vi "Measurement Logic.vi"() -> ()   [LabVIEW 2022 SP3, in "Single Tone - Digital Mic.lvlib"]
uses:
  Single Tone - Digital Mic.lvlib
  <vilib>/Plug-In SDKs/Measurements/Measure Call Context/Measure Call Context.lvclass
  Measurement Configuration.ctl
  shared/measurements/controls/lowpass filter.ctl
  shared/measurements/controls/weighting filter.ctl
  shared/measurements/controls/highpass filter.ctl
  shared/measurements/controls/measurement units.ctl
  Measurement Results.ctl
  <vilib>/addons/_NISVFA/_Generation/Signal Generation/SV Signal/sv_System Timing Model.ctl
  shared/Stop Variable Action.ctl
  <vilib>/PDM Acquisition Toolkit/host/Classes/Tasks/PDM Tasks/Controls/Acquisition Mode.ctl
  <vilib>/PDM Acquisition Toolkit/shared/controls/clock mode.ctl
  shared/measurements/controls/audio filter settings.ctl
  shared/measurements/controls/single tone microphone measurement settings.ctl
  shared/measurements/controls/units settings - mic.ctl
  <vilib>/DAQmx/read.llb/DAQmx Read (Analog Wfm 1Chan NSamp).vi
  <vilib>/DAQmx/write.llb/DAQmx Write (Analog Wfm 1Chan NSamp).vi
  <vilib>/addons/_NISVFA/_Generation/Signal Generation/SV Sinusoid/SV Sinusoid.lvclass
  C:/Program Files/NI/LVAddons/nisvt/1/vi.lib/addons/_NISVFA/_Generation/Signal Generation/SV Signal/SV Signal.lvclass
  <vilib>/addons/_NISVFA/_Generation/Signal Generation/SV Sinusoid/Configure Sine.vi
  <vilib>/DAQmx/create/channels.llb/DAQmx Create Channel (AO-Voltage-Basic).vi
  <vilib>/DAQmx/configure/timing.llb/DAQmx Timing (Sample Clock).vi
  <vilib>/DAQmx/configure/events/hardwareSignals.llb/DAQmx Export Signal (Most Signals).vi
  <vilib>/addons/_NISVFA/_Generation/Signal Generation/SV Signal/Write Sample Rate.vi
  <vilib>/addons/_NISVFA/_Generation/Signal Generation/SV Signal/Write System Timing Model.vi
  <vilib>/addons/_NISVFA/_Generation/Signal Generation/SV Signal/Write Ramp Parameters.vi
  <vilib>/DAQmx/create/channels.llb/DAQmx Create Channel (AI-Sound Pressure-Microphone).vi
  <vilib>/Waveform/WDTOps.llb/WDT Waveform Duration DBL.vi
  <vilib>/DAQmx/configure/trigger.llb/DAQmx Start Trigger (Digital Edge).vi
  <vilib>/DAQmx/miscellaneous.llb/DAQmx Fill In Error Info.vi
  <vilib>/Waveform/WDTOps.llb/WDT Get Waveform Subset DBL.vi
  <vilib>/addons/_NISVFA/_Generation/Signal Generation/SV Signal/SV Signal.lvclass
  <resource>/objmgr/daqmx.rc
  shared/combined digital api/Combo Digital Audio API.lvlib
  <vilib>/PDM Acquisition Toolkit/host/Classes/Tasks/PDM Tasks/PDM Task.lvclass
  <vilib>/PDM Acquisition Toolkit/shared/PDM Shared.lvlib
panel:
  out "calculated microphone sensitivity (dBFS)":dbl
  out "measurement results":T1={"channel name"="Empty", "frequency (Hz)"=0.0, "amplitude (Pa RMS)"=0.0, "amplitude (dBSPL)"=0.0, "microphone sensitivity (dBFS)"=0.0, "SNR"=0.0, "THD+N"=0.0, "THD"=0.0, "wfm - dt"=0.0, "wfm - data"=[0.0], "fft - f0"=0.0, "fft - df"=0.0, "fft - data"=[0.0], "ref mic wfm - dt"=0.0, "ref mic wfm - data"=[0.0]}
  in  "measurement configuration":T2={"digital channel list"="Lorem ipsum dolor sit", "input cfg file"="", "digital mic sensitivity (dBFS)"=1.2, "ref mic channel"="7821\\PCMo 0", "ref mic sensitivity (mV/Pa)"=32.0, "output channel"="7821\\PCMo 0", "signal frequency"=64.0, "output level (dBSPL)"=-32.0, "output voltage ratio"=-64.0, "lowpass filter"=enum."No filter", "weighting filter"=enum."A-weighting", "highpass filter"=enum."AC", "band start"=1.0, "band stop"=1.0, "min measurement cycles"=20, "min measurement time (s)"=0.1, "min settling cycles"=0, "min settling time (s)"=0.0, "SNR units"=enum."dB", "THD+N units"=enum."dB", "THD units"=enum."dB"} {"output voltage ratio" format="%#_g Pa/V"; "signal frequency" format="%#_13g"; "digital mic sensitivity (dBFS)" format="%#_13g"}
  out "measure call context out":refnum<class "Measure Call Context.lvclass">
  in  "measure call context in":refnum<class "Measure Call Context.lvclass">
  out "error out":errorcluster
  in  "error in":errorcluster
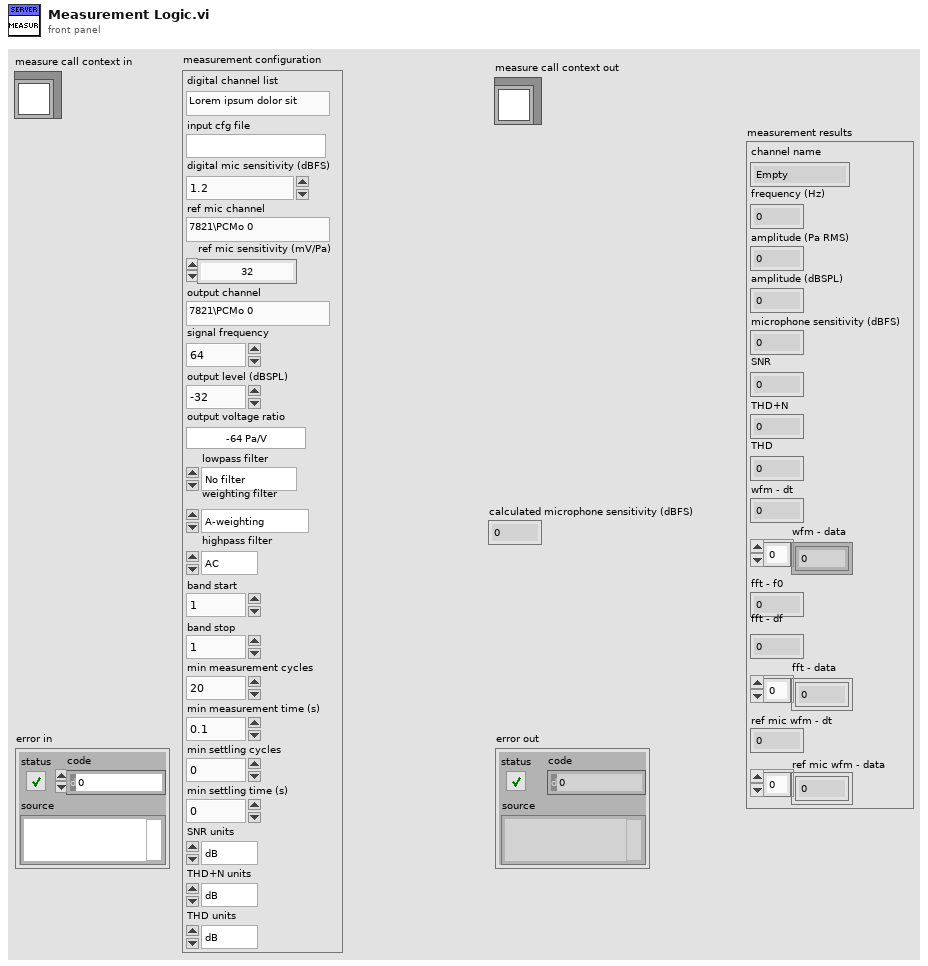
[diagram p1: front panel]
types:
  T1 = typedef "Single Tone - Digital Mic.lvlib/Measurement Results.ctl" = cluster{"channel name":string, "frequency (Hz)":dbl, "amplitude (Pa RMS)":dbl, "amplitude (dBSPL)":dbl, "microphone sensitivity (dBFS)":dbl, "SNR":dbl, "THD+N":dbl, "THD":dbl, "wfm - dt":dbl, "wfm - data":dbl[], "fft - f0":dbl, "fft - df":dbl, "fft - data":dbl[], "ref mic wfm - dt":dbl, "ref mic wfm - data":dbl[]}
  T2 = typedef "Single Tone - Digital Mic.lvlib/Measurement Configuration.ctl" = cluster{"digital channel list":string, "input cfg file":string, "digital mic sensitivity (dBFS)":dbl, "ref mic channel":string, "ref mic sensitivity (mV/Pa)":dbl, "output channel":string, "signal frequency":dbl, "output level (dBSPL)":dbl, "output voltage ratio":dbl, "lowpass filter":T3, "weighting filter":T4, "highpass filter":T5, "band start":dbl, "band stop":dbl, "min measurement cycles":u32, "min measurement time (s)":dbl, "min settling cycles":u32, "min settling time (s)":dbl, "SNR units":T6, "THD+N units":T6, "THD units":T6}
  T3 = typedef "lowpass filter.ctl" = enum32{"No filter", "AES17 20kHz", "AES17 40kHz"}
  T4 = typedef "weighting filter.ctl" = enum32{"Linear", "A-weighting", "B-weighting", "C-weighting"}
  T5 = typedef "highpass filter.ctl" = enum32{"DC", "AC"}
  T6 = typedef "measurement units.ctl" = enum32{"dB", "%", "x/y"}
  T7 = typedef "units settings - mic.ctl" = cluster{"SNR units":T6, "THD+N units":T6, "THD units":T6}
  T8 = typedef "single tone microphone measurement settings.ctl" = cluster{"Band start":dbl, "Band stop":dbl, "Frequency":dbl}
  T9 = typedef "audio filter settings.ctl" = cluster{"weighting filter":T4, "highpass filter":T5, "lowpass filter ":T3}
  T10 = typedef "PDM Shared.lvlib/clock mode.ctl" = enum16{"divided clock", "DDS"}
  T11 = typedef "PDM Acquisition Class Library.lvlib/PDM Task.lvclass/Acquisition Mode.ctl" = enum16{"Finite", "Continuous"}
  T12 = typedef "Stop Variable Action.ctl" = enum16{"Reset", "Check", "Stop"}
  T13 = typedef "SV Signal.lvclass/sv_System Timing Model.ctl" = i64
  T14 = cluster{"profile":enum16{"Linear", "Half cosine"}, "durations [s]":cluster{"ramp-up":dbl, "transition":dbl, "ramp-down":dbl}}
  T15 = typedef "Combo Digital Audio API.lvlib/task.ctl" = cluster{"task ref":u64, "audio type":T16, "sample rate":dbl}
  T16 = typedef "input type.ctl" = enum32{"Digital Serial", "PDM"}
  T17 = typedef "single tone microphone measurements.ctl" = cluster{"channel":string, "frequency (Hz)":dbl, "amplitude (Pa rms)":dbl, "amplitude (dBSPL)":dbl, "SNR":dbl, "THD+N":dbl, "THD":dbl, "phase (deg)":dbl}
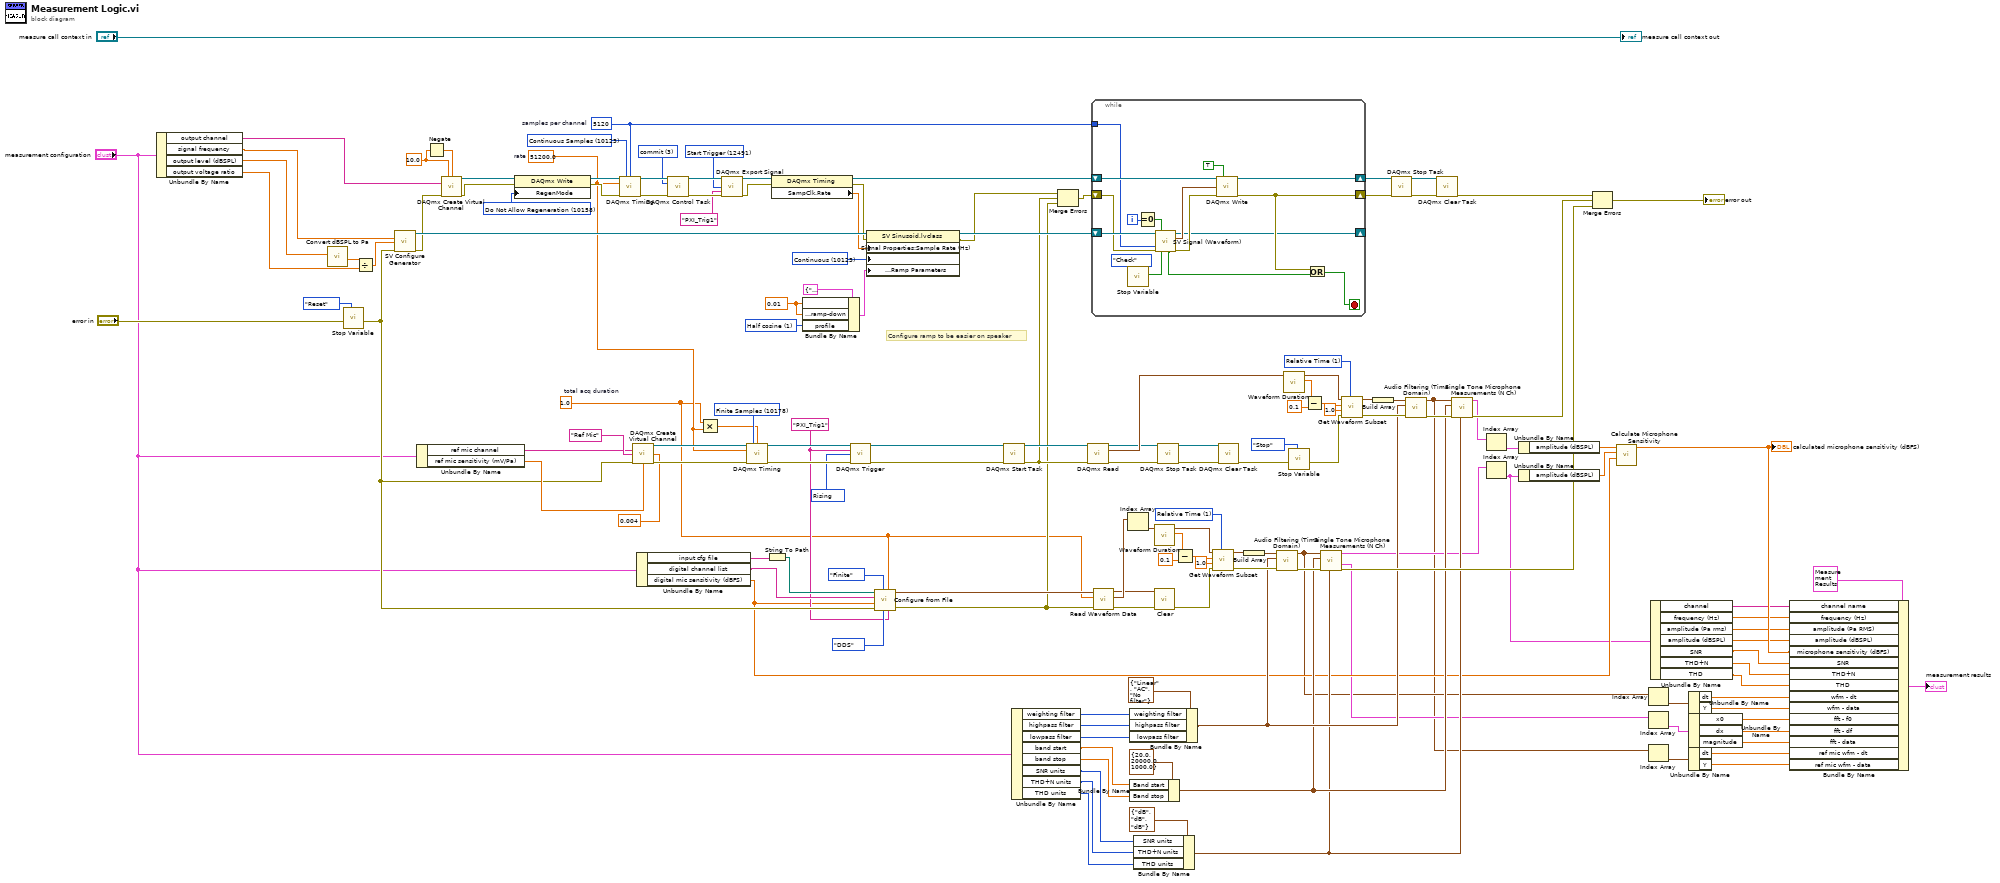
[diagram p0: block diagram]
diagram:
  w62 = u16 1 items=["Samples", "Relative Time"] ("start/duration format")
  w1 = 1.0  # total acq duration
  w91 = u16 1 items=["Samples", "Relative Time"] ("start/duration format")
  w103 = 10280 items=["Rising"=10280, "Falling"=10171] ("edge")
  w72 = "PXI_Trig1"
  w110 = 10178 items=["Finite Samples"=10178, "Continuous Samples"=10123] ("sample mode")
  w125 = 12491 items=["AI Convert Clock"=12484, "10MHz Reference Clock"=12536, "20MHz Timebase Clock"=12486, "Sample Clock"=12487, "Advance Trigger"=12488, "Reference Trigger"=12490, "Start Trigger"=12491, "Advance Complete Event"=12492, "AI Hold Complete Event"=12493, "Counter Output Event"=12494, "Change Detection Event"=12511, "Watchdog Timer Expired Event"=12512] ("signal")
  w130 = 3 items=["verify"=2, "reserve"=4, "commit"=3, "unreserve"=5, "abort"=6] ("action")
  w149 = 0.01 ("ramp duration")
  w147 = u16 1 items=["Linear", "Half cosine"] ("ramp profile")
  w141 = 10158 items=["Allow Regeneration"=10097, "Do Not Allow Regeneration"=10158] ("RegenMode")
  w144 = 10.0 ("maximum value")
  w111 = 5120  # samples per channel
  w145 = 10123 items=["Finite Samples"=10178, "Continuous Samples"=10123, "Hardware Timed Single Point"=12522] ("sample mode")
  w68 = 51200.0  # rate
  w146 = T13 10123 items=["Finite"=10178, "-"=-1, "Continuous"=10123, "-"=-2, "Settled"=110123, "Averaged"=210123, "Discrete Sweep"=310123, "Continuous Sweep"=410123] ("System Timing Model")
  # "Configure ramp to be easier on speaker"
  n1 = Unbundle By Name("measurement configuration") -> ("output channel"=w121:string, "signal frequency"=w120:dbl, "output level (dBSPL)"=w119:dbl, "output voltage ratio"=w118:dbl)
  n2 = call "Convert dBSPL to Pa.vi"("dB SPL"=w119) -> ("Pa pk"=w134:dbl)  [unwired: 9 in, 1 out]
  n3 = call "Stop Variable.vi"("action"=Stop_Variable_Action."Reset", "error in (no error)"="error in") -> ("error out"=w76:errorcluster)  [unwired: 8 in, 1 out]
  n4 = Divide(x=w134, y=w118) -> (x/y=w133:dbl)
  n5 = call-poly <vilib>:"SV Configure Generator.vi"("frequency (Hz)"=w120, "amplitude"=w133, "error in (no error)"=w76) -> ("signal configuration"=w151:refnum<class "SV Sinusoid.lvclass">, "error out"=w142:errorcluster)  [unwired: 11 in]
  n6 = Unbundle By Name("measurement configuration") -> ("ref mic channel"=w101:string, "ref mic sensitivity (mV/Pa)"=w100:dbl)
  n7 = Negate(x=w144) -> (-x=w143:dbl)
  n8 = call-poly <vilib>:"DAQmx Create Virtual Channel.vi"("maximum value"=w144, "minimum value"=w143, "physical channels"=w121, "error in"=w142) -> ("task out"=w140:refnum<k21>, "error out"=w138:errorcluster)  [unwired: 10 in]
  n9 = property class="DAQmx Write"(reference=w140, error in=w138, "RegenMode"=w141) -> (reference out=w139:refnum<k21>, error out=w137:errorcluster)
  n10 = call-poly <vilib>:"DAQmx Timing.vi"("task/channels in"=w139, "sample mode"=w145, "samples per channel"=w111, "rate"=w68, "error in"=w137) -> ("task out"=w132:refnum<k21>, "error out"=w131:errorcluster)  [unwired: 9 in]
  n11 = call-poly <vilib>:"DAQmx Create Virtual Channel.vi"("physical channels"=w101, "name to assign"="Ref Mic", "current excitation value"=0.004, "error in"=w76, "microphone sensitivity"=w100) -> ("task out"=w109:refnum<k21>, "error out"=w108:errorcluster)  [unwired: 9 in]
  n12 = Unbundle By Name("measurement configuration") -> ("input cfg file"=w78:string, "digital channel list"=w75:string, "digital mic sensitivity (dBFS)"=w27:dbl)
  n13 = call <vilib>:"DAQmx Control Task.vi"("task/channels in"=w132, "action"=w130, "error in"=w131) -> ("task out"=w129:refnum<k21>, "error out"=w128:errorcluster)  [unwired: 11 in]
  n14 = Multiply(x=w1, y=w68) -> (x*y=w69:dbl)
  n15 = call-poly <vilib>:"DAQmx Export Signal.vi"("task/channels in"=w129, "signal"=w125, "output terminal"="PXI_Trig1", "error in"=w128) -> ("task out"=w127:refnum<k21>, "error out"=w126:errorcluster)  [unwired: 10 in]
  n16 = call-poly <vilib>:"DAQmx Timing.vi"("task/channels in"=w109, "sample mode"=w110, "samples per channel"=w69, "rate"=w68, "error in"=w108) -> ("task out"=w107:refnum<k21>, "error out"=w105:errorcluster)  [unwired: 9 in]
  n17 = String To Path(string=w78) -> (path=w77:path)
  n18 = property class="DAQmx Timing"(reference=w127, error in=w126) -> (reference out=w113:refnum<k21>, error out=w135:errorcluster, "SampClk.Rate"=w136:dbl)
  n19 = Bundle By Name(cluster=T14 {"profile"=enum."Linear", "durations [s]"={"ramp-up"=0.0, "transition"=0.0, "ramp-down"=0.0}} ("Ramp Parameters:All Elements"), "durations [s].ramp-up"=w149, "durations [s].ramp-down"=w149, "profile"=w147) -> (w148:T14)
  n20 = call-poly <vilib>:"DAQmx Trigger.vi"("task/channels in"=w107, "source"=w72, "edge"=w103, "error in"=w105) -> ("task out"=w106:refnum<k21>, "error out"=w104:errorcluster)  [unwired: 10 in]
  n21 = property class="SV Sinusoid.lvclass"(reference=w151, error in=w135, "Signal Properties:Sample Rate (Hz)"=w136, "Signal Properties:System Timing Model"=w146, "Signal Properties:Ramps:Ramp Parameters"=w148) -> (reference out=w112:refnum<class "SV Sinusoid.lvclass">, error out=w97:errorcluster)
  n22 = call "Configure from File.vi"("digital trigger"=w72, "acq duration (s)"=w1, "clock mode"=clock_mode."DDS", "acquisition mode"=Acquisition_Mode."Finite", "error in (no error)"=w76, "microphone sensitivity (dBFS)"=w27, "channels"=w75, "file path"=w77) -> ("error out"=w70:errorcluster, "task"=w71:T15)  [unwired: 2 in]
  n23 = call <vilib>:"DAQmx Start Task.vi"("task/channels in"=w106, "error in"=w104) -> ("task out"=w89:refnum<k21>, "error out"=w88:errorcluster)  [unwired: 12 in]
  n24 = Unbundle By Name("measurement configuration") -> ("weighting filter"=w46:T4, "highpass filter"=w45:T5, "lowpass filter"=w44:T3, "band start"=w41:dbl, "band stop"=w40:dbl, "SNR units"=w35:T6, "THD+N units"=w34:T6, "THD units"=w33:T6)
  n25 = Merge Errors(w97, w88, w70) -> (w98:errorcluster)
  n26 = call-poly <vilib>:"DAQmx Read.vi"("task/channels in"=w89, "error in"=w88) -> ("task out"=w83:refnum<k21>, "data"=w90:waveform(dbl), "error out"=w50:errorcluster)  [unwired: 11 in]
  n27 = while {
    tunnel: w111 -> [w166]
    shift-right: [w164] -> w117
    shift-left: w113 -> [w168]
    shift-right: [w165] -> w116
    shift-left: w98 -> [w160]
    shift-right: [w159] -> _
    shift-left: w112 -> [w167]
    i -> [w156]
    stop <- w158 stop-if-true
    n28 = call "Stop Variable.vi"("action"=Stop_Variable_Action."Check") -> ("stop"=w154:bool)  [unwired: 9 in, 1 out]
    n29 = Equal To 0?(x=w156) -> (x = 0?=w157:bool)
    n30 = call-dynamic "SV Signal (Waveform).vi"("signal configuration"=w167, "reset"=w157, "samples"=w166, "error in (no error)"=w160, "stop"=w154) -> ("signal configuration"=w159:refnum<class "SV Sinusoid.lvclass">, "output waveform"=w162:waveform(dbl), "done"=w155:bool, "error out"=w163:errorcluster)  [unwired: 5 in, 2 out]
    n31 = call-poly <vilib>:"DAQmx Write.vi"("task/channels in"=w168, "auto start"=TRUE, "data"=w162, "error in"=w163) -> ("task out"=w164:refnum<k21>, "error out"=w165:errorcluster)  [unwired: 9 in, 1 out]
    n32 = Or(x=w165, y=w155) -> (x .or. y?=w158:bool)
  }
  n33 = call "Read Waveform Data.vi"("error in (no error)"=w70, "acq duration (s)"=w1, "task"=w71) -> ("error out"=w54:errorcluster, "waveforms"=w59:waveform(dbl)[], "task"=w53:T15)  [unwired: 6 in]
  n34 = Index Array(array=w59) -> (element=w60:waveform(dbl))  [unwired: 1 in]
  n35 = Bundle By Name(cluster=T9 {"weighting filter"=enum."Linear", "highpass filter"=enum."AC", "lowpass filter "=enum."No filter"} ("filter settings"), "weighting filter"=w46, "highpass filter"=w45, "lowpass filter"=w44) -> (w39:T9)
  n36 = Bundle By Name(cluster=T8 {"Band start"=20.0, "Band stop"=20000.0, "Frequency"=1000.0} ("measurement settings"), "Band start"=w41, "Band stop"=w40) -> (w38:T8)
  n37 = Bundle By Name(cluster=T7 {"SNR units"=enum."dB", "THD+N units"=enum."dB", "THD units"=enum."dB"} ("units settings"), "SNR units"=w35, "THD+N units"=w34, "THD units"=w33) -> (w36:T7)
  n38 = call-poly <vilib>:"Waveform Duration.vi"("waveform in"=w60) -> ("duration"=w67:dbl, "waveform out"=w63:waveform(dbl))  [unwired: 8 in, 1 out]
  n39 = call "Clear.vi"("error in (no error)"=w54, "task"=w53) -> ("error out"=w52:errorcluster)  [unwired: 9 in]
  n40 = call <vilib>:"DAQmx Stop Task.vi"("task/channels in"=w83, "error in"=w50) -> ("task out"=w87:refnum<k21>, "error out"=w86:errorcluster)  [unwired: 12 in]
  n41 = Subtract(x=w67, y=0.1) -> (x-y=w64:dbl)
  n42 = call-poly <vilib>:"Get Waveform Subset.vi"("start/duration format"=w62, "error in (no error)"=w52, "duration"=1.0, "start samples/time"=w64, "waveform in"=w63) -> ("error out"=w56:errorcluster, "waveform out"=w61:waveform(dbl))  [unwired: 1 in, 2 out]
  n43 = call <vilib>:"DAQmx Clear Task.vi"("task in"=w87, "error in"=w86) -> ("error out"=w84:errorcluster)  [unwired: 13 in]
  n44 = Build Array(w61) -> (w22:waveform(dbl)[])
  n45 = call "Audio Filtering (Time Domain).vi"("waveforms"=w22, "filter settings"=w39, "error in"=w56) -> ("time domain"=w20:waveform(dbl)[], "error out"=w55:errorcluster)  [unwired: 6 in]
  n46 = call-poly <vilib>:"Waveform Duration.vi"("waveform in"=w90) -> ("duration"=w96:dbl, "waveform out"=w92:waveform(dbl))  [unwired: 8 in, 1 out]
  n47 = call "Stop Variable.vi"("action"=Stop_Variable_Action."Stop", "error in (no error)"=w84) -> ("error out"=w49:errorcluster)  [unwired: 8 in, 1 out]
  n48 = Subtract(x=w96, y=0.1) -> (x-y=w93:dbl)
  n49 = call "Single Tone Microphone Measurements (N Ch).vi"("units settings"=w36, "error in"=w55, "measurement settings"=w38, "waveforms"=w20) -> ("error out"=w51:errorcluster, "spectra"=w21:cluster{"x0":dbl, "dx":dbl, "magnitude":dbl[]}[], "measurements"=w29:T17[])  [unwired: 4 in, 1 out]
  n50 = call-poly <vilib>:"Get Waveform Subset.vi"("start/duration format"=w91, "error in (no error)"=w49, "duration"=1.0, "start samples/time"=w93, "waveform in"=w92) -> ("error out"=w58:errorcluster, "waveform out"=w79:waveform(dbl))  [unwired: 1 in, 2 out]
  n51 = Build Array(w79) -> (w80:waveform(dbl)[])
  n52 = call <vilib>:"DAQmx Stop Task.vi"("task/channels in"=w117, "error in"=w116) -> ("task out"=w115:refnum<k21>, "error out"=w114:errorcluster)  [unwired: 12 in]
  n53 = call "Audio Filtering (Time Domain).vi"("waveforms"=w80, "filter settings"=w39, "error in"=w58) -> ("time domain"=w13:waveform(dbl)[], "error out"=w57:errorcluster)  [unwired: 6 in]
  n54 = call <vilib>:"DAQmx Clear Task.vi"("task in"=w115, "error in"=w114) -> ("error out"=w82:errorcluster)  [unwired: 13 in]
  n55 = call "Single Tone Microphone Measurements (N Ch).vi"("units settings"=w36, "error in"=w57, "measurement settings"=w38, "waveforms"=w13) -> ("error out"=w48:errorcluster, "measurements"=w32:T17[])  [unwired: 4 in, 2 out]
  n56 = Index Array(array=w32) -> (element=w31:T17)  [unwired: 1 in]
  n57 = Index Array(array=w29) -> (element=w9:T17)  [unwired: 1 in]
  n58 = Unbundle By Name(w31) -> ("amplitude (dBSPL)"=w30:dbl)
  n59 = Unbundle By Name(w9) -> ("amplitude (dBSPL)"=w28:dbl)
  n60 = Merge Errors(w82, w48, w51) -> (→"error out":errorcluster)
  n61 = call "Calculate Microphone Sensitivity.vi"("microphone sensitivity (dBFS)"=w27, "measured sound level (dBSPL)"=w28, "reference sound level (dBSPL)"=w30) -> ("calculated microphone sensitivity (dBFS)"=w10:dbl)  [unwired: 8 in]
  "calculated microphone sensitivity (dBFS)" <- w10
  n62 = Index Array(array=w20) -> (element=w24:waveform(dbl))  [unwired: 1 in]
  n63 = Index Array(array=w21) -> (element=w23:cluster{"x0":dbl, "dx":dbl, "magnitude":dbl[]})  [unwired: 1 in]
  n64 = Index Array(array=w13) -> (element=w14:waveform(dbl))  [unwired: 1 in]
  n65 = Unbundle By Name(w9) -> ("channel"=w8:string, "frequency (Hz)"=w7:dbl, "amplitude (Pa rms)"=w6:dbl, "amplitude (dBSPL)"=w5:dbl, "SNR"=w4:dbl, "THD+N"=w3:dbl, "THD"=w2:dbl)
  n66 = Unbundle By Name(w24) -> ("dt"=w19:dbl, "Y"=w18:dbl[])
  n67 = Unbundle By Name(w23) -> ("x0"=w17:dbl, "dx"=w16:dbl, "magnitude"=w15:dbl[])
  n68 = Unbundle By Name(w14) -> ("dt"=w12:dbl, "Y"=w11:dbl[])
  n69 = Bundle By Name(cluster=T1 {"channel name"="Empty", "frequency (Hz)"=0.0, "amplitude (Pa RMS)"=0.0, "amplitude (dBSPL)"=0.0, "microphone sensitivity (dBFS)"=0.0, "SNR"=0.0, "THD+N"=0.0, "THD"=0.0, "wfm - dt"=0.0, "wfm - data"=[0.0], "fft - f0"=0.0, "fft - df"=0.0, "fft - data"=[0.0], "ref mic wfm - dt"=0.0, "ref mic wfm - data"=[0.0]} ("measurement results"), "channel name"=w8, "frequency (Hz)"=w7, "amplitude (Pa RMS)"=w6, "amplitude (dBSPL)"=w5, "microphone sensitivity (dBFS)"=w10, "SNR"=w4, "THD+N"=w3, "THD"=w2, "wfm - dt"=w19, "wfm - data"=w18, "fft - f0"=w17, "fft - df"=w16, "fft - data"=w15, "ref mic wfm - dt"=w12, "ref mic wfm - data"=w11) -> (→"measurement results":T1)
  "measure call context out" <- "measure call context in"
